vi "Bind to Type - Non Serializable Class - Returns LabVIEW Object.vi"() -> ()   [LabVIEW 2017, in "JSON Serializable Binder Tests.lvlib"]
uses:
  JSON Serializable Binder Tests.lvlib
  JSON Serializable Binder/JSON Serializable Binder.lvclass
  <vilib>/addons/_JKI Toolkits/Caraya/classes/Assert/Assert Equal Value and Type_Variant.vi
  <vilib>/addons/_JKI Toolkits/Caraya/classes/Test/Test.lvclass
  <vilib>/addons/_JKI Toolkits/Caraya/classes/Assert/Assert.lvclass
panel:
  out "error out":errorcluster
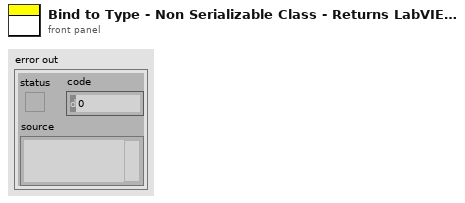
[diagram p1: front panel]
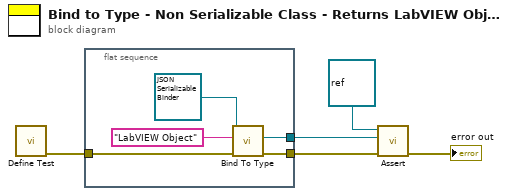
[diagram p0: block diagram]
diagram:
  n1 = call <vilib>:"Define Test.vi"() -> ("error out"=w5:errorcluster)  [unwired: 11 in]
  n2 = flat-sequence {
    tunnel: w5 -> [w10]
    tunnel: [w7] -> w3
    tunnel: [w6] -> w2
    frame #0 {
      n3 = call-dynamic "Bind To Type.vi"("error in (no error)"=w10, "Type Name"="LabVIEW Object", "JSON Serializable Binder in"=refnum<class "JSON Serializable Binder.lvclass"> refnum ("JSON Serializable Binder.lvclass")) -> ("error out"=w7:errorcluster, "Type"=w6:refnum<class>)  [unwired: 6 in, 1 out]
    }
  }
  n4 = call-poly <vilib>:"Assert.vi"("error in (no error)"=w3, "Y"=w2, "X"=refnum<class> refnum ("target class")) -> ("error out"=→"error out":errorcluster)  [unwired: 8 in]
